vi "NewClientMessage.vi"(8 "error in (no error)":errorcluster, 10 "Message from client":string, 11 "TCP_Client_Window in":refnum<class "TCP_Client_Window.lvclass">) -> (0 "error out":errorcluster, 3 "TCP_Client_Window out":refnum<class "TCP_Client_Window.lvclass">)   [LabVIEW 2023, in "TCP_Client_Window.lvlib" / "TCP_Client_Window.lvclass"]
uses:
  TCP_Client_Window.lvclass
  TCP_Client_Window.lvclass/TCP_Client_Window.ctl
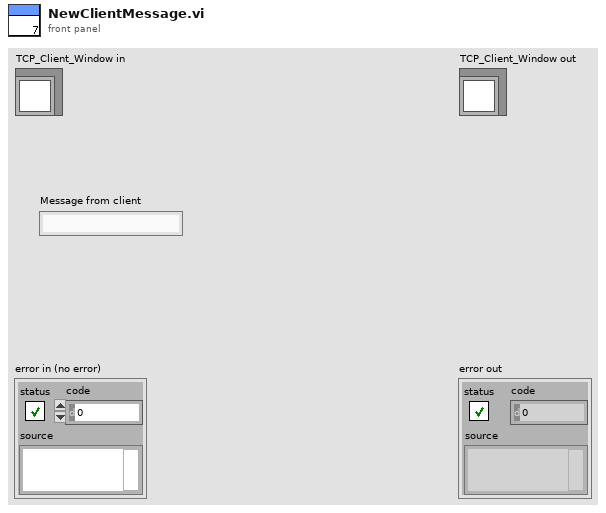
[diagram p1: front panel]
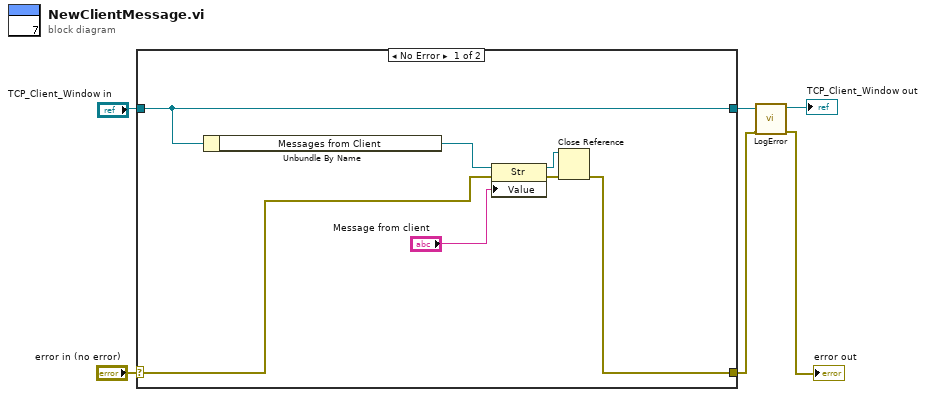
[diagram p0: block diagram]
diagram:
  n1 = case shown="No Error" "error in (no error)" {
    selector: "error in (no error)" -> [w10 w15]
    tunnel: [w7 w15] -> w2
    tunnel: [w13 w14] -> w4
    tunnel: "TCP_Client_Window in" -> [w13 w14]
    frame No Error {
      n2 = Unbundle By Name(w13) -> ("Messages from Client"=w12:refnum<vi>)
      n3 = property class="Str"(reference=w12, error in=w10, "Value"="Message from client") -> (reference out=w8:refnum<vi>, error out=w9:errorcluster)
      n4 = Close Reference(reference=w8, error in (no error)=w9) -> (error out=w7:errorcluster)
    }
    frame Error {
    }
  }
  n5 = call "LogError.vi"("error in (no error)"=w2, "TCP_Client_Window in"=w4) -> ("error out"=→"error out":errorcluster, "TCP_Client_Window out"=→"TCP_Client_Window out":refnum<class "TCP_Client_Window.lvclass">)  [unwired: 8 in]
